vi "20T_Go_To_Zero.vi"(8 "error in (no error)":errorcluster, 10 "20T Control":T1={"Clamp"=TRUE, "Switch Heater"=TRUE, "Go to Zero"=TRUE, "Go to Set"=FALSE, "Go to Hold"=FALSE, "Field Setpoint (T)"=3.4572, "Rate Setpoint (T/min)"=0.0, "Set Rate"=FALSE, "Activate lambda control"=FALSE, "Set lambda NV"=FALSE, "lambda NV  SP"=3.4572} {"lambda NV  SP" format="%.1f"; "Rate Setpoint (T/min)" format="%6_5f"; "Field Setpoint (T)" format="%#4_5f"}, 11 "Mercury Reference In":T2) -> (0 "error out":errorcluster)   [LabVIEW 2019]
uses:
  Equipment/Mercury iXX/Public/Controls/Mercury Reference.ctl
  Equipment/Mercury iXX/Public/Controls/Comms Transport Layer.ctl
  Equipment/Mercury iXX/Private/Controls/Query Dynamic Reference.ctl
  Monitor Communication/Gustav/20T_Control.ctl
  Global/Global Variables/Data_Display_global.vi
  Equipment/Mercury iXX/Public/Libraries/Magnet/Open/Open Magnet Device.vi
  Monitor Communication/sub-vis/20T_Open_Queue.vi
  Monitor Communication/sub-vis/20T_Queue_Commands.vi
  Equipment/Mercury iXX/Mercury iXX.lvlib
  Equipment/Mercury iXX/Public/Libraries/Magnet.lvlib
panel:
  # "20 T"
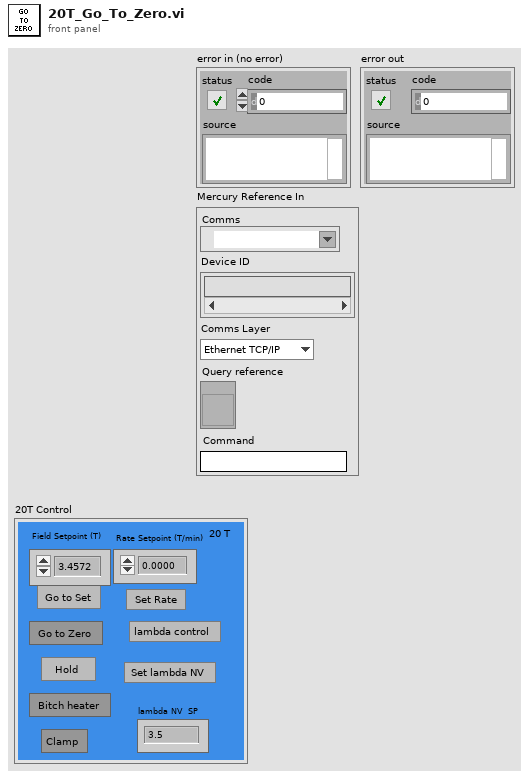
[diagram p1: front panel]
types:
  T1 = typedef "20T_Control.ctl" = cluster{"Clamp":bool, "Switch Heater":bool, "Go to Zero":bool, "Go to Set":bool, "Go to Hold":bool, "Field Setpoint (T)":dbl, "Rate Setpoint (T/min)":dbl, "Set Rate":bool, "Activate lambda control":bool, "Set lambda NV":bool, "lambda NV  SP":dbl}
  T2 = typedef "Mercury iXX.lvlib/Mercury Reference.ctl" = cluster{"Comms":refnum<visa-resource-name>, "Device ID":string[], "Comms Layer":T3, "Command":string, "Query reference":T4}
  T3 = typedef "Mercury iXX.lvlib/Comms Transport Layer.ctl" = enum16{"Ethernet TCP/IP", "USB", "ISOBus - RS-232", "GPIB"}
  T4 = typedef "Mercury iXX.lvlib/Query Dynamic Reference.ctl" = refnum<vi>
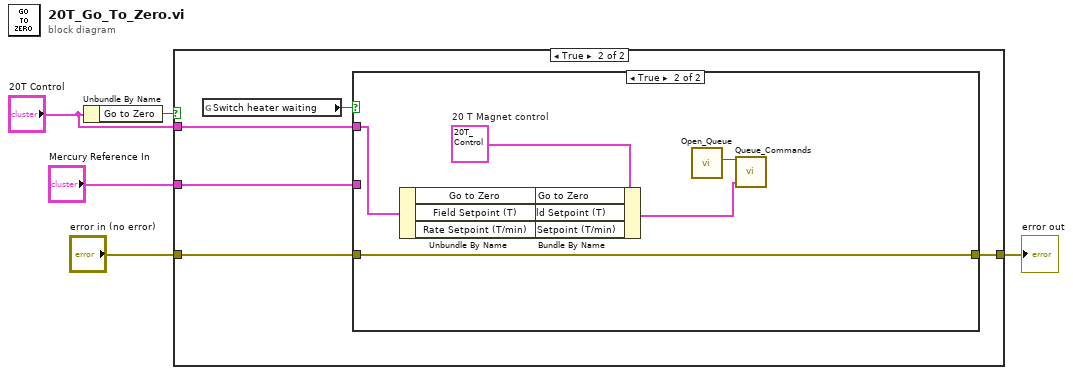
[diagram p0: block diagram]
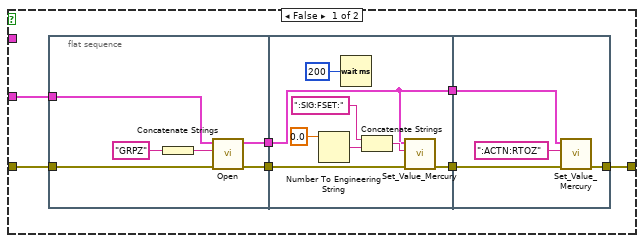
[diagram p3: hidden frame]
diagram:
  n1 = Unbundle By Name("20T Control") -> ("Go to Zero"=w3:bool)
  n2 = case shown="True" w3 {
    tunnel: "Mercury Reference In" -> [_ w11]
    tunnel: "error in (no error)" -> [w6 w10]
    tunnel: [w6 w7] -> w2
    tunnel: "20T Control" -> [_ w8]
    frame False {
    }
    frame True {
      n3 = global read "Data_Display_global.vi" "Switch heater waiting"() -> (w9:bool)
      n4 = case shown="True" w9 {
        tunnel: w11 -> [w14 _]
        tunnel: w10 -> [w13 w44]
        tunnel: [w12 w44] -> w7
        tunnel: w8 -> [_ w37]
        frame False {
          n5 = flat-sequence {
            tunnel: w14 -> [w22]
            tunnel: w13 -> [w21]
            tunnel: [w20] -> w18
            tunnel: [w19] -> w17
            tunnel: w18 -> [w25]
            tunnel: [w26] -> w16
            tunnel: w17 -> [w27]
            tunnel: [w25] -> w15
            tunnel: w16 -> [w35]
            tunnel: [w34] -> w12
            tunnel: w15 -> [w33]
            frame #0 {
              n6 = Concatenate Strings("GRPZ" ("Device Identifier")) -> (w24:string)
              n7 = call-poly "Open.vi"("error in (no error)"=w21, "Device Identifier"=w24, "Mercury Reference In"=w22) -> ("error out"=w19:errorcluster, "Mercury Reference Out"=w20:T2)  [unwired: 1 in, 6 out]
            }
            frame #1 {
              n8 = Number To Engineering String(4:0.0) -> (0:w32:string)  [unwired: 3 in]
              n9 = Wait (ms)(milliseconds to wait=200) -> ()  [unwired: 1 out]
              n10 = Concatenate Strings(":SIG:FSET:", w32) -> (w30:string)
              n11 = call "Set_Value_Mercury.vi"("error in"=w27, "Noun(s)"=w30, "Mercury Reference In"=w25) -> ("error out"=w26:errorcluster)  [unwired: 7 in, 1 out]
            }
            frame #2 {
              n12 = call "Set_Value_Mercury.vi"("error in"=w35, "Noun(s)"=":ACTN:RTOZ", "Mercury Reference In"=w33) -> ("error out"=w34:errorcluster)  [unwired: 7 in, 1 out]
            }
          }
        }
        frame True {
          w42 = T1 {"Clamp"=FALSE, "Switch Heater"=FALSE, "Go to Zero"=FALSE, "Go to Set"=FALSE, "Go to Hold"=FALSE, "Field Setpoint (T)"=3.4572, "Rate Setpoint (T/min)"=0.0, "Set Rate"=FALSE, "Activate lambda control"=FALSE, "Set lambda NV"=FALSE, "lambda NV  SP"=3.4572}  # 20 T Magnet control
          n13 = Unbundle By Name(w37) -> ("Go to Zero"=w40:bool, "Field Setpoint (T)"=w39:dbl, "Rate Setpoint (T/min)"=w38:dbl)
          n14 = Bundle By Name(cluster=w42, "Go to Zero"=w40, "Field Setpoint (T)"=w39, "Rate Setpoint (T/min)"=w38) -> (w41:T1)
          n15 = call-poly "Open_Queue.vi"() -> ("queue out"=w43:refnum<queue>)  [unwired: 10 in, 1 out]
          n16 = call-poly "Queue_Commands.vi"("20T Control (in)"=w41, "20T Queue"=w43) -> ()  [unwired: 1 in, 1 out]
        }
      }
    }
  }
  "error out" <- w2
